vi "control_lasers_and_SMs_timing.vi"() -> ()   [LabVIEW 2021]
uses:
  <vilib>/DAQmx/write.llb/DAQmx Write (Analog 1D DBL NChan 1Samp).vi
  <vilib>/DAQmx/create/channels.llb/DAQmx Create Channel (AO-Voltage-Basic).vi
  <vilib>/DAQmx/configure/timing.llb/DAQmx Timing (Sample Clock).vi
  <vilib>/DAQmx/miscellaneous.llb/DAQmx Fill In Error Info.vi
panel:
  in  "Y1 (-10-10V) 3":dbl
  in  "X1 (-10-10V) 3":dbl
  in  "Blanking (0-10v) 3":dbl=10.0
  in  "445 (0-10v) 3":dbl
  in  "Y1 (-10-10V) 2":dbl
  in  "X1 (-10-10V) 2":dbl
  in  "Blanking (0-10v) 2":dbl=10.0
  in  "445 (0-10v) 2":dbl
  in  "Y1 (-10-10V)":dbl
  in  "X1 (-10-10V)":dbl
  in  "Blanking (0-10v)":dbl=10.0
  in  "445 (0-10v)":dbl
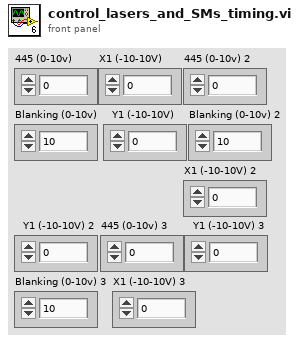
[diagram p1: front panel]
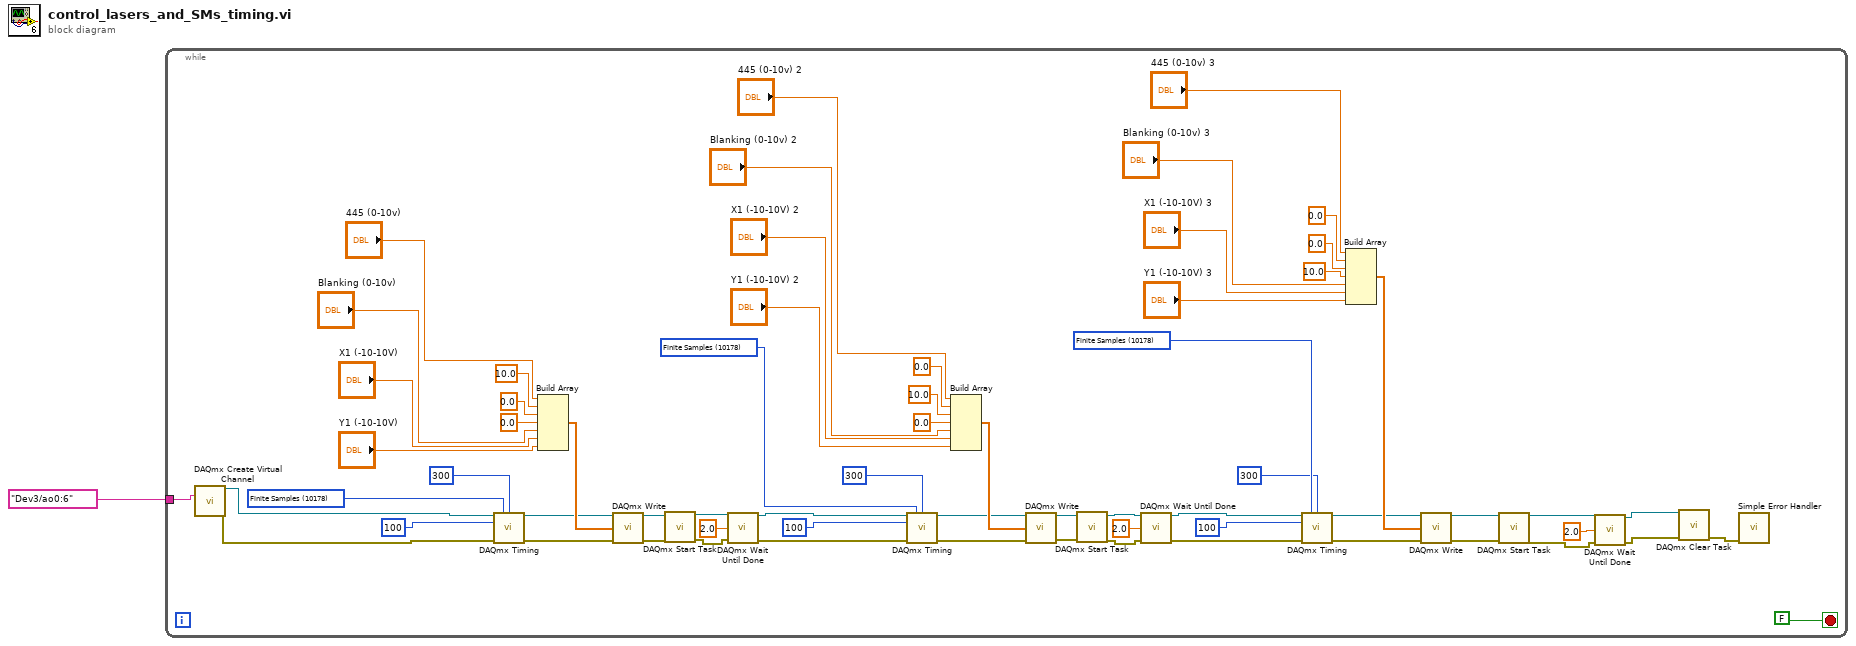
[diagram p0: block diagram]
diagram:
  n1 = while {
    tunnel: tag "Dev3/ao0:6" ("physical channels") -> [w16]
    stop <- FALSE stop-if-true
    w28 = 10178 items=["Finite Samples"=10178, "Continuous Samples"=10123, "Hardware Timed Single Point"=12522] ("sample mode")
    w41 = 10178 items=["Finite Samples"=10178, "Continuous Samples"=10123, "Hardware Timed Single Point"=12522] ("sample mode")
    w46 = 10178 items=["Finite Samples"=10178, "Continuous Samples"=10123, "Hardware Timed Single Point"=12522] ("sample mode")
    n2 = call-poly <vilib>:"DAQmx Create Virtual Channel.vi"("physical channels"=w16) -> ("task out"=w15:refnum<k21>, "error out"=w14:errorcluster)  [unwired: 13 in]
    n3 = call-poly <vilib>:"DAQmx Timing.vi"("task/channels in"=w15, "sample mode"=w46, "samples per channel"=300, "rate"=100, "error in"=w14) -> ("task out"=w43:refnum<k21>, "error out"=w42:errorcluster)  [unwired: 9 in]
    n4 = Build Array("445 (0-10v)", 10.0, 0.0, 0.0, "Blanking (0-10v)", "X1 (-10-10V)", "Y1 (-10-10V)") -> (w62:dbl[])
    n5 = call-poly <vilib>:"DAQmx Write.vi"("task/channels in"=w43, "data"=w62, "error in"=w42) -> ("task out"=w13:refnum<k21>, "error out"=w12:errorcluster)  [unwired: 10 in, 1 out]
    n6 = call <vilib>:"DAQmx Start Task.vi"("task/channels in"=w13, "error in"=w12) -> ("task out"=w11:refnum<k21>, "error out"=w10:errorcluster)  [unwired: 12 in]
    n7 = call <vilib>:"DAQmx Wait Until Done.vi"("task/channels in"=w11, "timeout (sec)"=2.0, "error in"=w10) -> ("task out"=w23:refnum<k21>, "error out"=w22:errorcluster)  [unwired: 11 in]
    n8 = call-poly <vilib>:"DAQmx Timing.vi"("task/channels in"=w23, "sample mode"=w41, "samples per channel"=300, "rate"=100, "error in"=w22) -> ("task out"=w39:refnum<k21>, "error out"=w38:errorcluster)  [unwired: 9 in]
    n9 = Build Array("445 (0-10v) 2", 0.0, 10.0, 0.0, "Blanking (0-10v) 2", "X1 (-10-10V) 2", "Y1 (-10-10V) 2") -> (w55:dbl[])
    n10 = call-poly <vilib>:"DAQmx Write.vi"("task/channels in"=w39, "data"=w55, "error in"=w38) -> ("task out"=w9:refnum<k21>, "error out"=w6:errorcluster)  [unwired: 10 in, 1 out]
    n11 = call <vilib>:"DAQmx Start Task.vi"("task/channels in"=w9, "error in"=w6) -> ("task out"=w8:refnum<k21>, "error out"=w7:errorcluster)  [unwired: 12 in]
    n12 = call <vilib>:"DAQmx Wait Until Done.vi"("task/channels in"=w8, "timeout (sec)"=2.0, "error in"=w7) -> ("task out"=w20:refnum<k21>, "error out"=w19:errorcluster)  [unwired: 11 in]
    n13 = call-poly <vilib>:"DAQmx Timing.vi"("task/channels in"=w20, "sample mode"=w28, "samples per channel"=300, "rate"=100, "error in"=w19) -> ("task out"=w26:refnum<k21>, "error out"=w25:errorcluster)  [unwired: 9 in]
    n14 = Build Array("445 (0-10v) 3", 0.0, 0.0, 10.0, "Blanking (0-10v) 3", "X1 (-10-10V) 3", "Y1 (-10-10V) 3") -> (w36:dbl[])
    n15 = call-poly <vilib>:"DAQmx Write.vi"("task/channels in"=w26, "data"=w36, "error in"=w25) -> ("task out"=w5:refnum<k21>, "error out"=w3:errorcluster)  [unwired: 10 in, 1 out]
    n16 = call <vilib>:"DAQmx Start Task.vi"("task/channels in"=w5, "error in"=w3) -> ("task out"=w4:refnum<k21>, "error out"=w2:errorcluster)  [unwired: 12 in]
    n17 = call <vilib>:"DAQmx Wait Until Done.vi"("task/channels in"=w4, "timeout (sec)"=2.0, "error in"=w2) -> ("task out"=w65:refnum<k21>, "error out"=w64:errorcluster)  [unwired: 11 in]
    n18 = call <vilib>:"DAQmx Clear Task.vi"("task in"=w65, "error in"=w64) -> ("error out"=w66:errorcluster)  [unwired: 13 in]
    n19 = call <vilib>:"Simple Error Handler.vi"("error in (no error)"=w66) -> ()  [unwired: 4 in, 5 out]
  }
